vi "createCommunicator.vi"(8 "error in (no error)":errorcluster, 11 "Boot in":refnum<class "Boot.lvclass">) -> (0 "error out":errorcluster, 2 "Communicator":refnum<class "Communicator.lvclass">, 3 "Boot out":refnum<class "Boot.lvclass">)   [LabVIEW 2016, in "Boot.lvclass"]
uses:
  Boot.lvclass
  Communicator/Communicator/Communicator.lvclass
  Communicator/M1M3SAL/M1M3SAL.lvclass
  D:/Code/ts_M1M3Support/Communicator/Communicator/Communicator.lvclass
  Communicator/M1M3SAL/M1M3SAL.lvclass/M1M3SAL.ctl
  Boot.lvclass/Boot.ctl
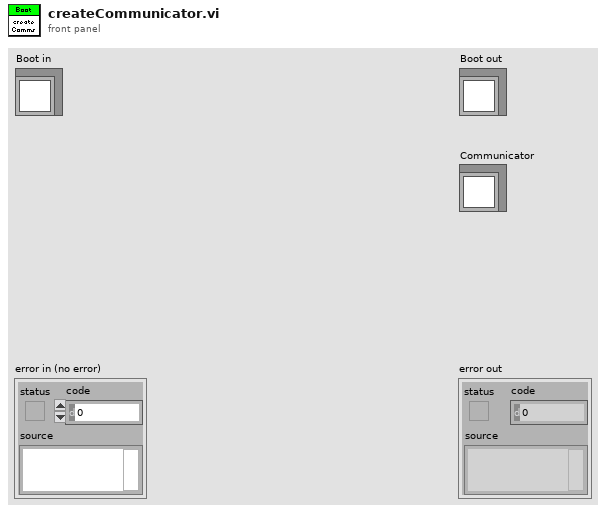
[diagram p1: front panel]
types:
  T1 = typedef "M1M3Communicator.lvlib/M1M3SALSettings.ctl" = cluster{"IPAddress":string, "Port":u16, "StartupScript":string}
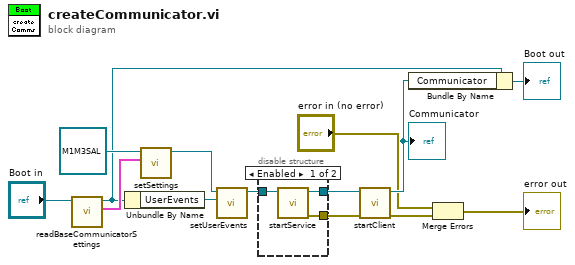
[diagram p0: block diagram]
diagram:
  n1 = call "readBaseCommunicatorSettings.vi"("Boot in"="Boot in") -> ("M1M3SALSettings"=w7:T1, "Boot out"=w6:refnum<class "Boot.lvclass">)  [unwired: 8 in, 1 out]
  n2 = Unbundle By Name(w6) -> ("UserEvents"=w9:refnum<class "UserEvents.lvclass">)
  n3 = call "setSettings.vi"("Settings"=w7, "M1M3SAL in"=refnum<class "M1M3SAL.lvclass"> refnum ("M1M3Communicator.lvlib:M1M3SAL.lvclass")) -> ("M1M3SAL out"=w13:refnum<class "M1M3SAL.lvclass">)  [unwired: 9 in]
  n4 = call "setUserEvents.vi"("UserEvents"=w9, "M1M3SAL in"=w13) -> ("M1M3SAL out"=w12:refnum<class "M1M3SAL.lvclass">)  [unwired: 9 in]
  n5 = disable-structure shown="Enabled" {
    disable-tunnel: w12 -> [w17 w18]
    disable-tunnel: [w16 w18] -> w11
    disable-tunnel: [w15 _] -> w10
    frame Enabled {
      n6 = call-dynamic "startService.vi"("M1M3SAL in"=w17) -> ("error out"=w15:errorcluster, "M1M3SAL out"=w16:refnum<class "M1M3SAL.lvclass">)  [unwired: 9 in]
    }
    frame Disabled {
    }
  }
  n7 = call-dynamic "startClient.vi"("error in (no error)"=w10, "M1M3SAL in"=w11) -> ("error out"=w2:errorcluster, "M1M3SAL out"=w4:refnum<class "M1M3SAL.lvclass">)  [unwired: 8 in]
  "Communicator" <- w4
  n8 = Bundle By Name(cluster=w6, "Communicator"=w4) -> (→"Boot out":refnum<class "Boot.lvclass">)
  n9 = Merge Errors("error in (no error)", w2) -> (→"error out":errorcluster)
